vi "Get Grid Radius.vi"(8 "error in (no error)":errorcluster, 10 "Origin Coords":T3, 11 "Control Ref Cluster":T1) -> (0 "error out":errorcluster, 2 "Dup Origin Coords":T3, 3 "Dup Control Ref Cluster":T1, 4 "Radius Array":i16[](array[numeric]))   [LabVIEW 2017, in "2D Compass.lvclass"]
uses:
  <vilib>/Math Plots/2D Math Plots/2D Compass/2D Compass/2D Compass.lvclass
  <vilib>/Utility/miscctls.llb/LVPoint32TypeDef.ctl
  <vilib>/Math Plots/2D Math Plots/2D Plot/Action String/2DMathPlot Ctrl Act Cluster.ctl
  <vilib>/Math Plots/2D Math Plots/2D Plot/Action String/2DMathPlot State Class.ctl
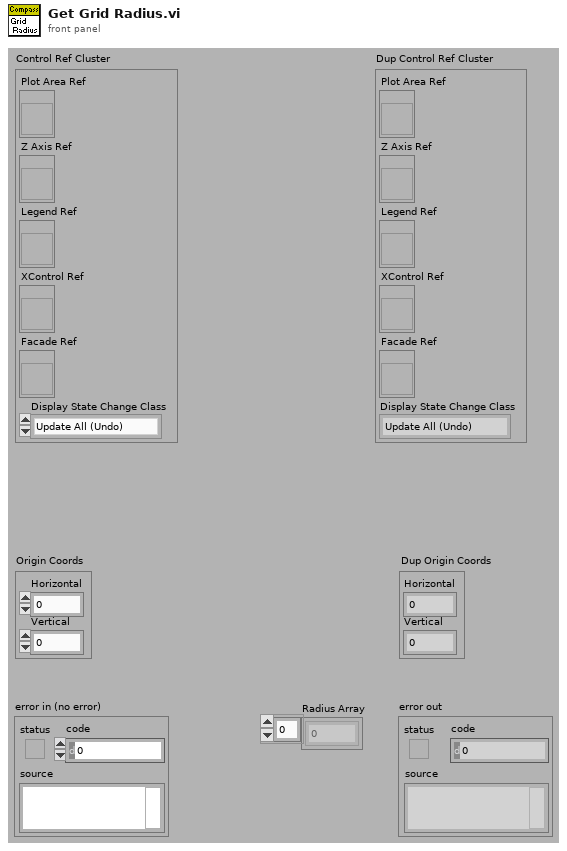
[diagram p1: front panel]
types:
  T1 = typedef "2DMathPlot Ctrl Act Cluster.ctl" = cluster{"Plot Area Ref":refnum<vi>, "Z Axis Ref":refnum<vi>, "Legend Ref":refnum<vi>, "XControl Ref":refnum<vi>, "Facade Ref":refnum<vi>, "Display State Change Class":T2}
  T2 = typedef "2DMathPlot State Class.ctl" = enum16{"Update All (Undo)", "Update General", "Update Appearance", "Update Format", "Update Scale", "Update Marker", "Update Cursor", "None"}
  T3 = typedef "LVPoint32TypeDef.ctl" = cluster{"Horizontal":i32, "Vertical":i32}
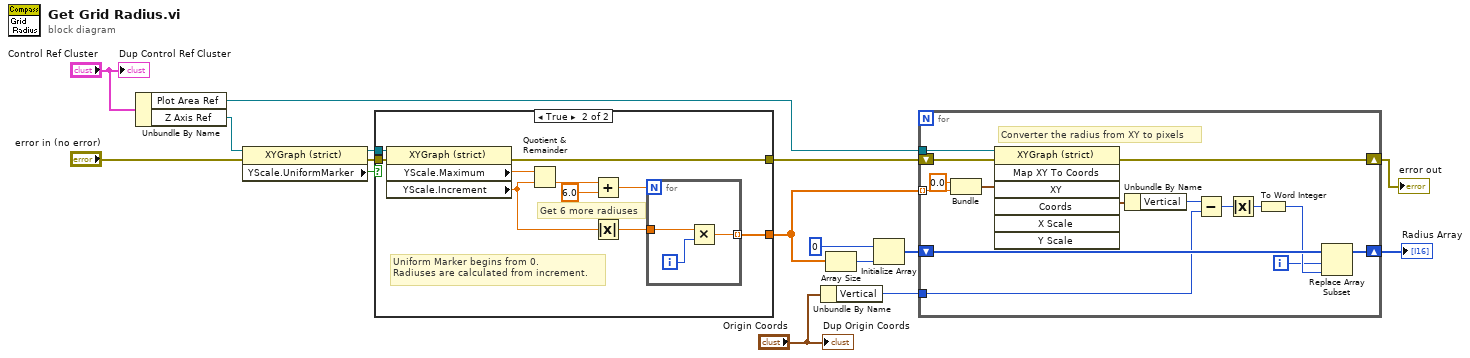
[diagram p0: block diagram]
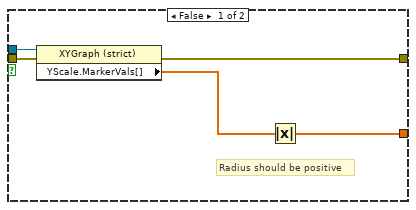
[diagram p2: hidden frame]
diagram:
  n1 = Unbundle By Name("Control Ref Cluster") -> ("Plot Area Ref"=w1:refnum<vi>, "Z Axis Ref"=w2:refnum<vi>)
  n2 = property class="XYGraph (strict)"(reference=w2, error in="error in (no error)") -> (reference out=w15:refnum<vi>, error out=w14:errorcluster, "YScale.UniformMarker"=w8:bool)
  n3 = case shown="True" w8 {
    tunnel: w15 -> [w21 w31]
    tunnel: w14 -> [w20 w30]
    tunnel: [w17 w25] -> w6
    tunnel: [w18 w27] -> w11
    frame False {
      # "Radius should be positive"
      n4 = property class="XYGraph (strict)"(reference=w21, error in=w20) -> (error out=w18:errorcluster, "YScale.MarkerVals[]"=w19:dbl[])  [unwired: 1 out]
      n5 = Absolute Value(x=w19) -> (abs(x)=w17:dbl[])
    }
    frame True {
      # "Get 6 more radiuses"
      # "Uniform Marker begins from 0.\nRadiuses are calculated from increment."
      n6 = property class="XYGraph (strict)"(reference=w31, error in=w30) -> (error out=w27:errorcluster, "YScale.Maximum"=w29:dbl, "YScale.Increment"=w26:dbl)  [unwired: 1 out]
      n7 = Quotient & Remainder(x=w29, y=w26) -> (floor(x/y)=w28:dbl)  [unwired: 1 out]
      n8 = Add(x=w28, y=6.0 ("x")) -> (x+y=w24:dbl)
      n9 = Absolute Value(x=w26) -> (abs(x)=w22:dbl)
      n10 = for {
        N: w24 -> [_]
        tunnel: w22 -> [w34]
        tunnel: [w32] -> w25 mode=indexing
        i -> [w33]
        n11 = Multiply(x=w34, y=w33) -> (x*y=w32:dbl)
      }
    }
  }
  n12 = Unbundle By Name("Origin Coords") -> ("Vertical"=w10:i32)
  n13 = Array Size(array=w6) -> (size(s)=w5:i32)
  n14 = Initialize Array(i16 0, w5) -> (w4:i16[])
  n15 = for {
    tunnel: w6 -> [w47] mode=indexing
    shift-right: [w49] -> w16
    shift-left: w4 -> [w48]
    tunnel: w10 -> [w46]
    shift-right: [w44] -> w13
    shift-left: w11 -> [w45]
    tunnel: w1 -> [w35]
    i -> [w36]
    # "Converter the radius from XY to pixels"
    n16 = Bundle(0.0, w47) -> (w43:cluster{dbl, dbl})  [unwired: 1 out]
    n17 = invoke on="Invoke Node" class="XYGraph (strict)" method="Map XY To Coords"(reference=w35, error in=w45, "XY"=w43) -> (error out=w44:errorcluster, "Coords"=w42:T3)  [unwired: 4 in, 5 out]
    n18 = Unbundle By Name(w42) -> ("Vertical"=w41:i32)
    n19 = Subtract(x=w41, y=w46) -> (x-y=w39:i32)
    n20 = Absolute Value(x=w39) -> (abs(x)=w38:i32)
    n21 = To Word Integer(number=w38) -> (16bit integer=w37:i16)
    n22 = Replace Array Subset(array=w48, new element=w37, index=w36) -> (w49:i16[])
  }
  "Radius Array" <- w16
  "error out" <- w13
  "Dup Origin Coords" <- "Origin Coords"
  "Dup Control Ref Cluster" <- "Control Ref Cluster"
